vi "DAQ@AnalogOut__Parameter.vi"(1 "ParamterIn":string) -> (0 "ParamterOut":string)   [LabVIEW 2020]
panel:
  in  "Voltage":string(combo)
  in  "DAQName":string(combo)
  in  "Confirm":bool
  # "DAQ@AnalogOut $DAQ,$Voltage"
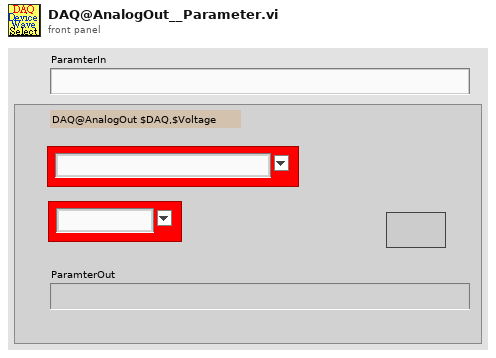
[diagram p1: front panel]
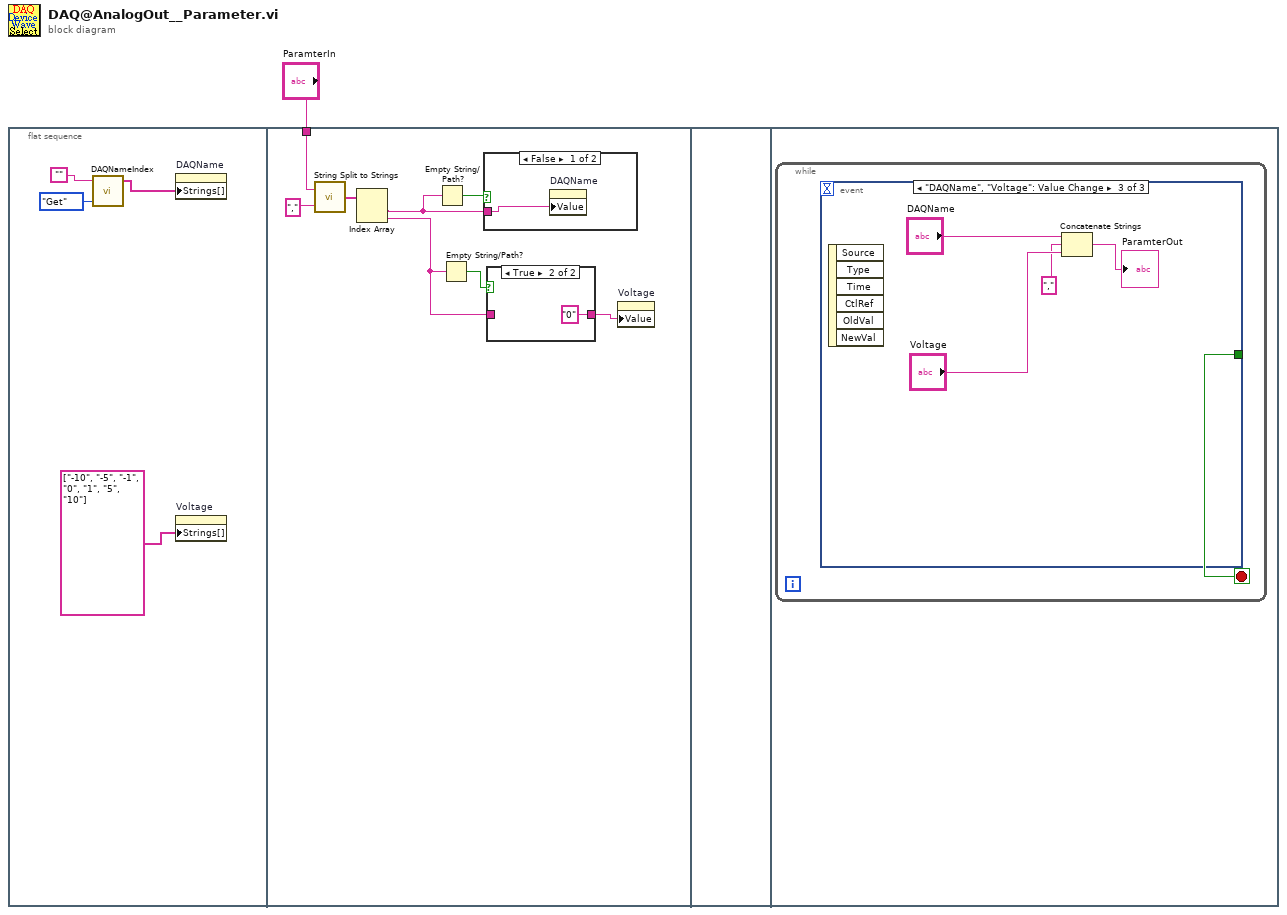
[diagram p0: block diagram]
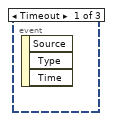
[diagram p4: hidden frame]
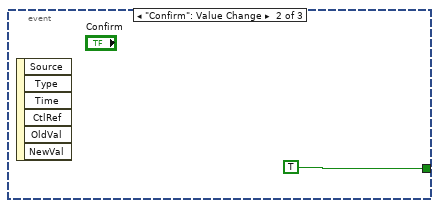
[diagram p5: hidden frame]
diagram:
  n1 = flat-sequence {
    tunnel: "ParamterIn" -> [w10]
    frame #0 {
      n2 = call "DAQNameIndex.vi"("OP"=enum16{"Get", "Update", "Init"}."Get", "DAQName"="") -> ("DAQList"=w3:string[])  [unwired: 1 in, 2 out]
      n3 = property on="DAQName" class="CmbBox"("Strings[]"=w3) -> ()  [unwired: 2 in, 2 out]
      n4 = property on="Voltage" class="CmbBox"("Strings[]"=string[] ["-10", "-5", "-1", "0", "1", "5", "10"] ("Strings []")) -> ()  [unwired: 2 in, 2 out]
    }
    frame #1 {
      n5 = call "String Split to Strings.vi"("search string/char (-)"=",", "String"=w10) -> ("Array"=w12:string[])
      n6 = Index Array(array=w12) -> (element #1=w9:string, element #2=w6:string)  [unwired: 2 in]
      n7 = Empty String/Path?(string/path=w9) -> (empty?=w13:bool)
      n8 = Empty String/Path?(string/path=w6) -> (empty?=w8:bool)
      n9 = case shown="False" w13 {
        tunnel: w9 -> [w16 _]
        frame False {
          n10 = property on="DAQName" class="CmbBox"("Value"=w16) -> ()  [unwired: 2 in, 2 out]
        }
        frame True {
        }
      }
      n11 = case shown="True" w8 {
        tunnel: [w14 "0" ("ParamterIn")] -> w7
        tunnel: w6 -> [w14 _]
        frame False {
        }
        frame True {
        }
      }
      n12 = property on="Voltage" class="CmbBox"("Value"=w7) -> ()  [unwired: 2 in, 2 out]
    }
    frame #2 {
    }
    frame #3 {
      n13 = while {
        stop <- w17 stop-if-true
        n14 = event shown="[2] \"DAQName\", \"Voltage\": Value Change" {
          selector: _ -> [_ _ _]
          dyn-events: _ -> [_ _ _]
          timeout: _ -> [_ _ _]
          tunnel: [_ TRUE _] -> w17
          event Timeout {
            n15 = event-data() -> ()  [unwired: 1 in, 3 out]
          }
          event "Confirm": Value Change {
            n16 = event-data() -> ()  [unwired: 1 in, 6 out]
          }
          event "DAQName", "Voltage": Value Change {
            n17 = event-data() -> ()  [unwired: 1 in, 6 out]
            n18 = Concatenate Strings("DAQName", ",", "Voltage") -> (→"ParamterOut":string)
          }
        }
      }
    }
  }
